vi "Validity Check.vi"(8 "error in (no error)":errorcluster, 11 "sentence":string) -> (0 "error out":errorcluster, 3 "valid sentence":bool)   [LabVIEW 2009]
doc: "Specifies whether the formatting of an NMEA sentence is valid."
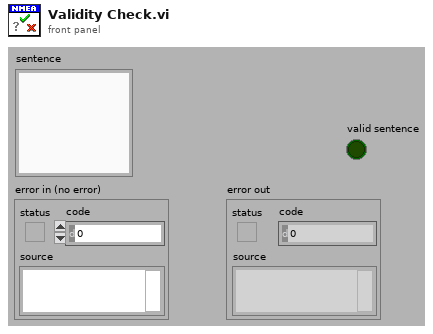
[diagram p1: front panel]
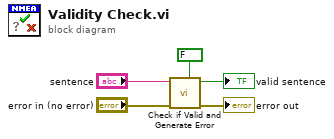
[diagram p0: block diagram]
diagram:
  n1 = call "Check if Valid and Generate Error.vi"("generate error if invalid (F)"=FALSE, "error in (no error)"="error in (no error)", "sentence"="sentence") -> ("error out"=→"error out":errorcluster, "valid sentence"=→"valid sentence":bool)  [unwired: 7 in]
